vi "Read Bias Voltage (V).vi"(11 "LCR Meter in":refnum<class "LCR Meter.lvclass">) -> (2 "Bias Voltage (V)":dbl, 3 "LCR Meter out":refnum<class "LCR Meter.lvclass">)   [LabVIEW 2020, in "LCR Meter.lvclass"]
uses:
  LCR Meter.lvclass
  LCR Meter.lvclass/LCR Meter.ctl
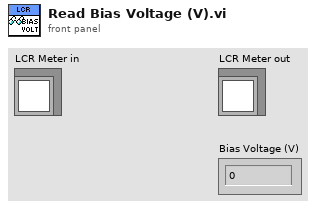
[diagram p1: front panel]
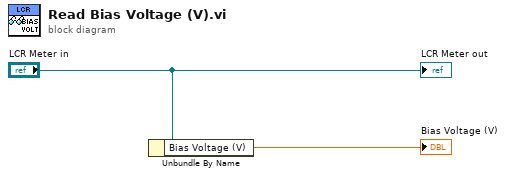
[diagram p0: block diagram]
diagram:
  n1 = Unbundle By Name("LCR Meter in") -> ("Bias Voltage (V)"=→"Bias Voltage (V)":dbl)
  "LCR Meter out" <- "LCR Meter in"
